vi "displayFrequency.vi"(0 "FrequencyViewer.lvclass":refnum<class "FrequencyViewer.lvclass">) -> (1 "Current Frequency":string, 2 "Current Frequency":dbl)   [LabVIEW 2009, in "Hardware.lvlib" / "frequencyCounters.lvlib" / "FrequencyViewer.lvclass"]
uses:
  FrequencyViewer.lvclass
  FrequencyViewer.lvclass/FrequencyViewer.ctl
panel:
  out "Waveform Chart":dbl[](graph)
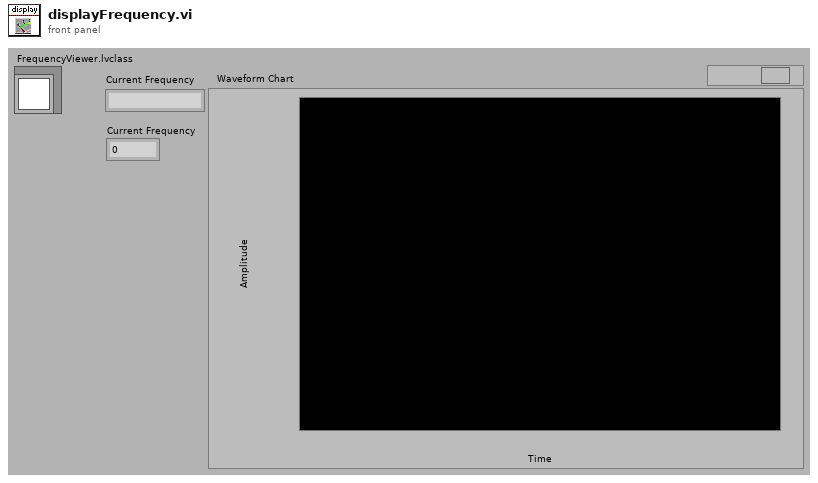
[diagram p1: front panel]
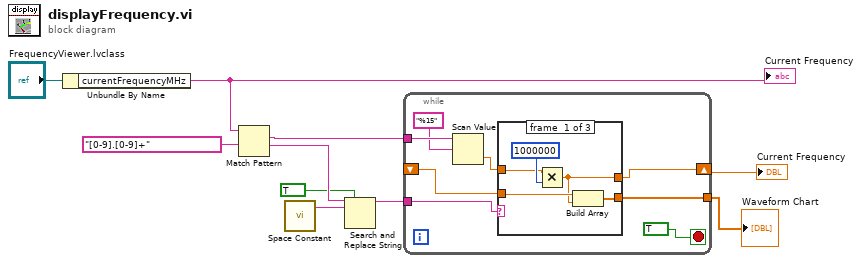
[diagram p0: block diagram]
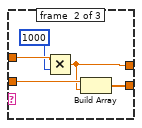
[diagram p2: hidden frame]
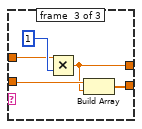
[diagram p3: hidden frame]
diagram:
  n1 = Unbundle By Name("FrequencyViewer.lvclass") -> ("currentFrequencyMHz"=w9:string)
  "Current Frequency" <- w9
  n2 = Match Pattern(string=w9, regular expression="[0-9].[0-9]+") -> (match substring=w5:string, after substring=w4:string)  [unwired: 1 in, 2 out]
  n3 = call <vilib>:"Space Constant.vi"() -> ("String"=w2:string)
  n4 = Search and Replace String(replace all?=TRUE, input string=w4, search string=w2) -> (result string=w3:string)  [unwired: 5 in, 3 out]
  n5 = while {
    shift-right: [w11] -> w6
    shift-left: _ -> [w15]
    tunnel: w5 -> [w17]
    tunnel: [w14] -> w7
    tunnel: w3 -> [w13]
    stop <- TRUE stop-if-true
    n6 = Scan Value(string=w17, format string="%15") -> (value=w12:dbl)  [unwired: 1 in, 1 out]
    n7 = case shown="\"kHz\"" w13 {
      tunnel: w15 -> [w21 w28 w32]
      tunnel: w12 -> [w22 w26 w30]
      tunnel: [w20 w27 w31] -> w14
      tunnel: [w19 w24 w29] -> w11
      frame #0 {
        n8 = Multiply(x=w22, y=1000000) -> (x*y=w19:dbl)
        n9 = Build Array(w21, w19) -> (w20:dbl[])
      }
      frame #1 {
        n10 = Multiply(x=w26, y=1000) -> (x*y=w24:dbl)
        n11 = Build Array(w28, w24) -> (w27:dbl[])
      }
      frame #2 {
        n12 = Multiply(x=w30, y=1) -> (x*y=w29:dbl)
        n13 = Build Array(w32, w29) -> (w31:dbl[])
      }
    }
  }
  "Waveform Chart" <- w7
  "Current Frequency" <- w6
